vi "BotSpeak_FILE SAVE.vi"(2 "file name":string="test.htm", 3 "HTML text":string="<!DOCTYPE html>\n<html>\n<body>\n\n<h1>My First Heading</h1>\n\n<p>My first paragraph.</p>\n\n</body>\n</html>\n", 4 "Bot Settings":T1) -> (0 "response":string="169.254.32.85", 1 "Bot Settings 2":T1)   [LabVIEW 2012]
doc: "Saves the desired \"HTML text\" to the RIO as the specified \"file name\"."
uses:
  <userlib>/BotSpeak/VIs/Direct/BotSpeak_Control.ctl
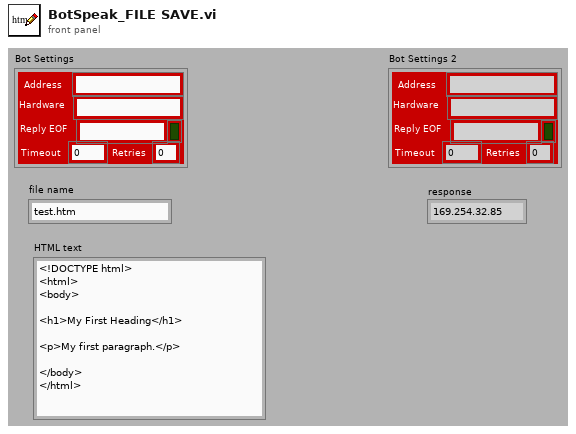
[diagram p1: front panel]
types:
  T1 = typedef "BotSpeak_Control.ctl" = cluster{"Address":string, "Reply EOF":string, "Hardware":string, "Retries":i8, "Timeout":i32, "Open?":bool}
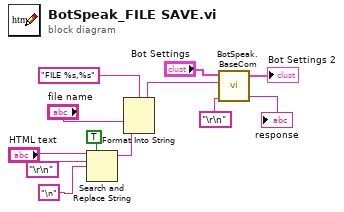
[diagram p0: block diagram]
diagram:
  n1 = Search and Replace String(replace all?=TRUE ("replace all? (F)"), input string="HTML text", search string="\r\n", replace string="\n" ("search string")) -> (result string=w10:string)  [unwired: 4 in, 3 out]
  n2 = Format Into String(format string="FILE %s,%s" ("command"), "file name", w10) -> (resulting string=w2:string)  [unwired: 2 in, 1 out]
  n3 = call <userlib>:"BotSpeak.BaseCom.vi"("Termination"="\r\n", "command"=w2, "Bot Settings in"="Bot Settings") -> ("response"=→"response":string, "Bot Settings out"=→"Bot Settings 2":T1)  [unwired: 2 in]
